vi "Method Elements.vi"(6 "Arduino In":cluster{"Error In":errorcluster, "LINX In":T1}, 7 "Potential Calibration":dbl[][](array[numeric])=[[1.0, 0.0, 5.4592, 5.4592]], 8 "Input--Scan Rate":cluster{"DE (V)":dbl, "Dt (s)":dbl}={"DE (V)"=1.0, "Dt (s)"=1.0} {"Dt (s)" format="%0.2f"; "DE (V)" format="%0.2f"}, 9 "Input--Timing":T9={"Duration (s)"=30.0, "Sample Rate (ms)"=100.0, "Frequency (mHz)"=1000.0, "Repeat n Times"=0}, 10 "Input--Potential":T8={"Ei (V)"=0.0, "Ef (V)"=1.0, "E1 (V)"=1.0, "E2 (V)"=-1.0, "Duty Cycle (%)"=50.0}, 11 "Element":T10(ring)) -> (3 "Output":T7, 4 "Arduino Out":cluster{"Error Out":errorcluster, "LINX Out":T1})   [LabVIEW 2022 SP3]
uses:
  <vilib>/MakerHub/LINX/Private/Type Defs/LINX Ref.ctl
  <vilib>/MakerHub/LINX/Private/Type Defs/Platform.ctl
  <vilib>/MakerHub/LINX/Private/Type Defs/Interface.ctl
  <vilib>/MakerHub/LINX/Private/Device/Type Defs/LINX Device Config.ctl
  <vilib>/MakerHub/LINX/Private/Device/Type Defs/TCP Config.ctl
  <vilib>/MakerHub/LINX/Private/Device/Type Defs/Channels.ctl
  <vilib>/Analysis/1siggen.llb/Ramp Pattern by Samples.vi
  <vilib>/Analysis/NI_AALBase.lvlib
  <vilib>/MakerHub/LINX/LMH-LINX.lvlib
  <vilib>/MakerHub/LINX/Private/Device/Device.lvlib
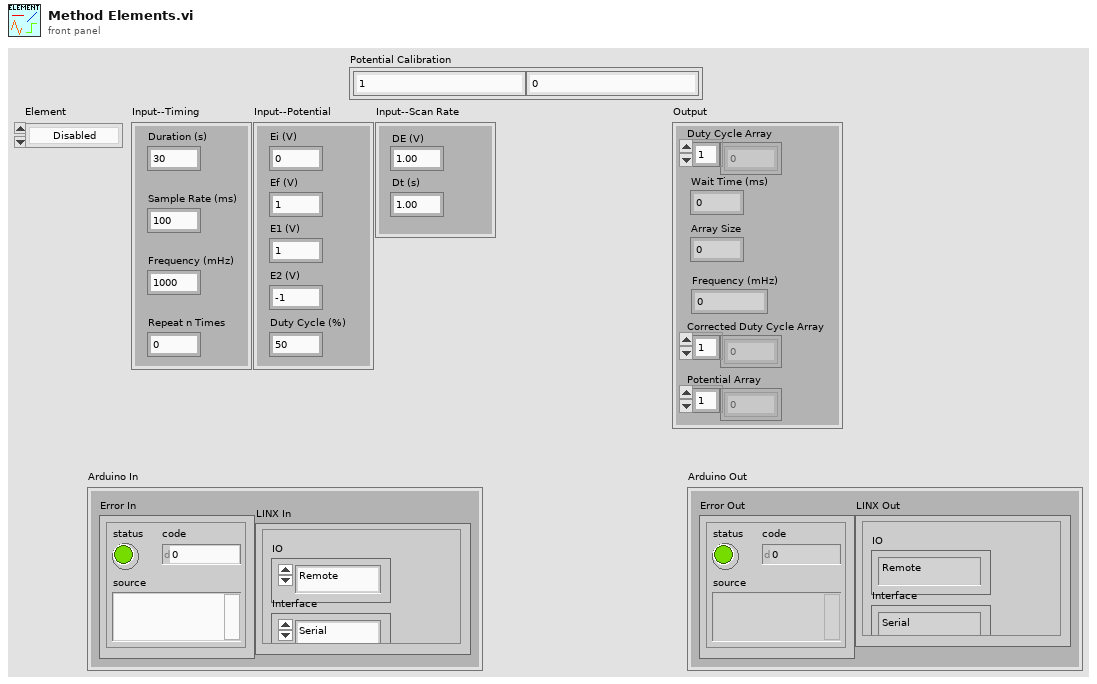
[diagram p1: front panel]
types:
  T1 = typedef "LMH-LINX.lvlib/LINX Ref.ctl" = cluster{"IO":T2, "Interface":T3, "LINX Device Config":T4}
  T2 = typedef "LMH-LINX.lvlib/Platform.ctl" = enum16{"Remote", "Local"}
  T3 = typedef "LMH-LINX.lvlib/Interface.ctl" = enum16{"Serial", "TCP"}
  T4 = typedef "LMH-LINX.lvlib/Device.lvlib/LINX Device Config.ctl" = cluster{"Interface":T3, "COM Port":refnum<visa-resource-name>, "TCP Configuration":T5, "Device Family":u8, "Device ID":u8, "Device Name":string, "TCP Ref":refnum<k5>, "Channels":T6}
  T5 = typedef "LMH-LINX.lvlib/Device.lvlib/TCP Config.ctl" = cluster{"IP Address":string, "Port":u16}
  T6 = typedef "LMH-LINX.lvlib/Channels.ctl" = cluster{"DI":u8[], "DO":u8[], "AI":u8[], "AO":u8[], "PWM":u8[], "QE":u8[], "UART":u8[], "I2C 2":u8[], "SPI":u8[], "CAN":u8[], "Servo":u8[], "AI Ref (V)":dbl, "AI Resolution (Bits)":u8, "AO Ref (V)":dbl, "AO Resolution (Bits)":u8}
  T7 = cluster{"Duty Cycle Array":dbl[], "Wait Time (ms)":dbl, "Array Size":i32, "Frequency (mHz)":dbl, "Corrected Duty Cycle Array":dbl[], "Potential Array":dbl[]}
  T8 = cluster{"Ei (V)":dbl, "Ef (V)":dbl, "E1 (V)":dbl, "E2 (V)":dbl, "Duty Cycle (%)":dbl}
  T9 = cluster{"Duration (s)":dbl, "Sample Rate (ms)":dbl, "Frequency (mHz)":dbl, "Repeat n Times":i32}
  T10 = enum16{"Disabled", "Potentiostatic", "Linear Ramp", "Staircase Ramp", "Triangle Wave", "Square Wave", "Staircase Wave", "Sine Wave"}
  T11 = cluster{dbl[], "Sample Rate (ms)":dbl, i32, "Frequency (mHz)":dbl, dbl[], "Ramp Pattern":dbl[]}
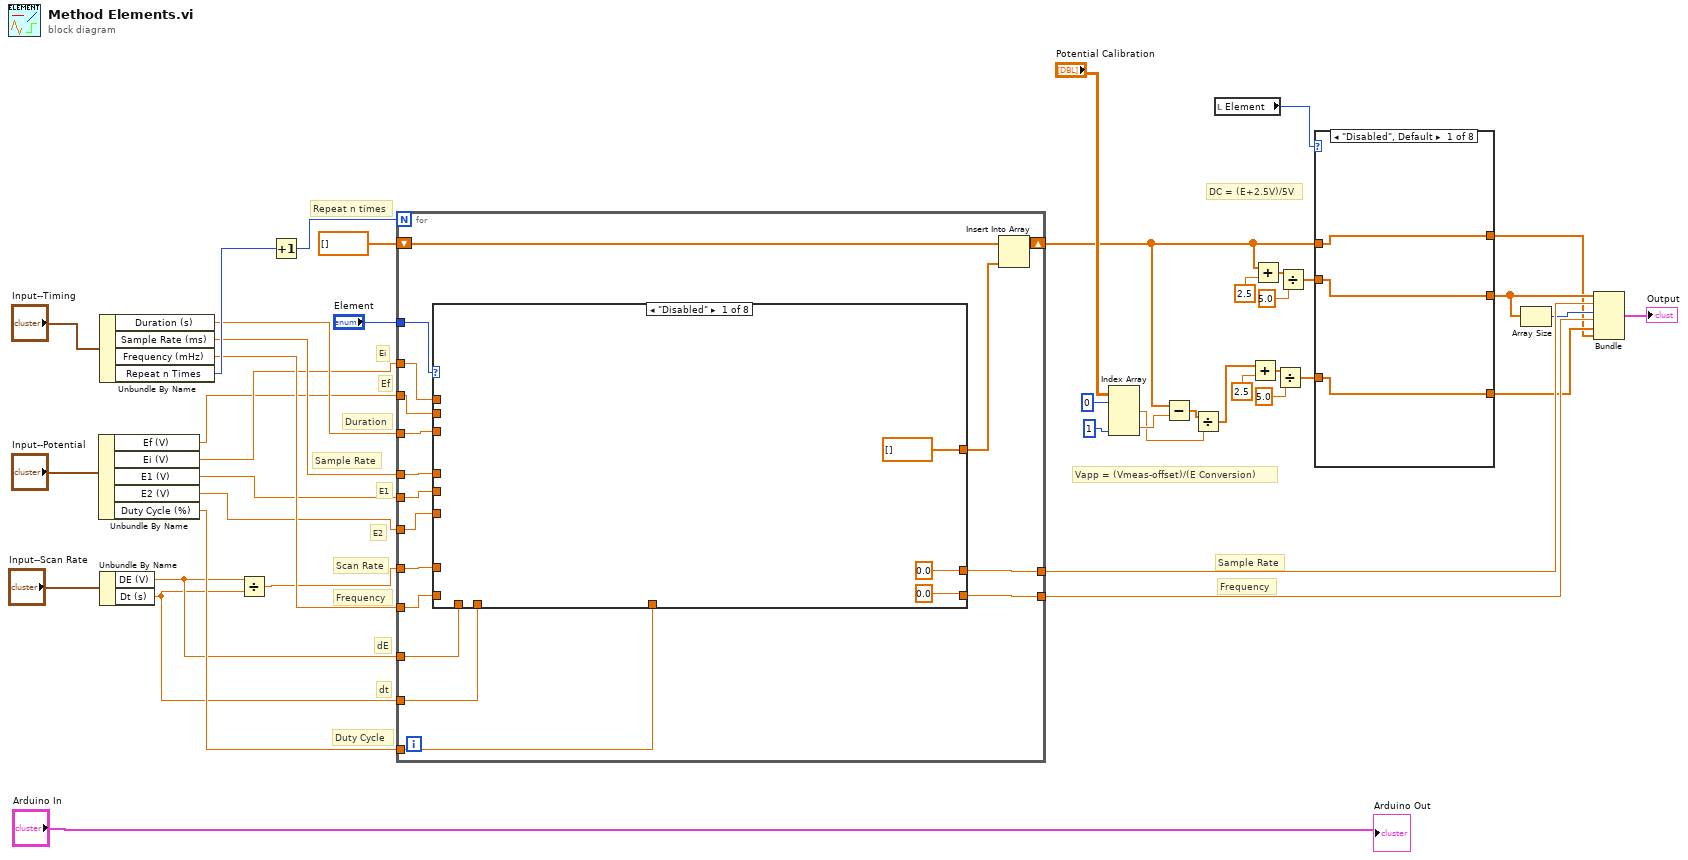
[diagram p0: block diagram]
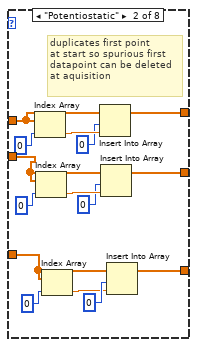
[diagram p2: hidden frame]
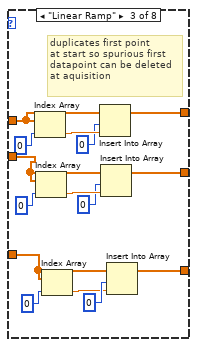
[diagram p3: hidden frame]
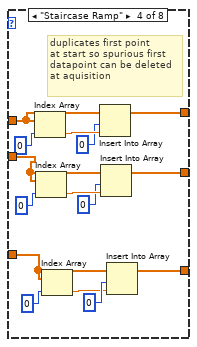
[diagram p4: hidden frame]
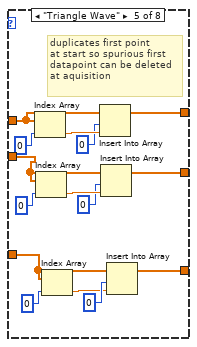
[diagram p5: hidden frame]
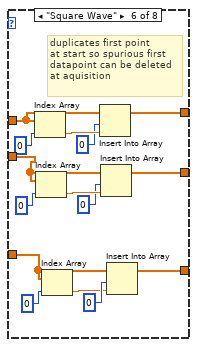
[diagram p6: hidden frame]
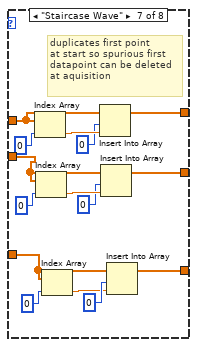
[diagram p7: hidden frame]
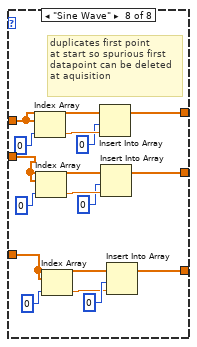
[diagram p8: hidden frame]
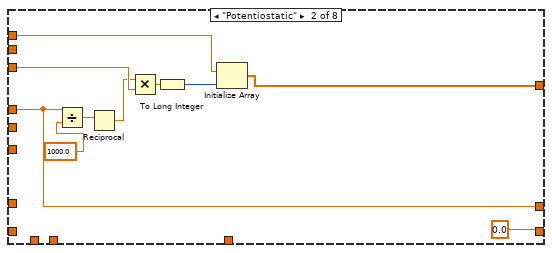
[diagram p9: hidden frame]
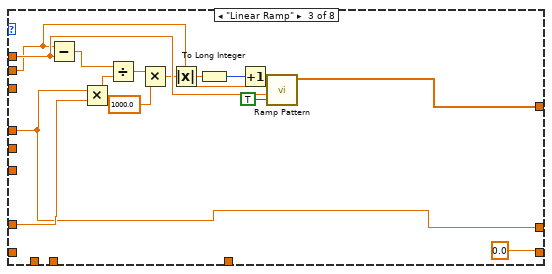
[diagram p10: hidden frame]
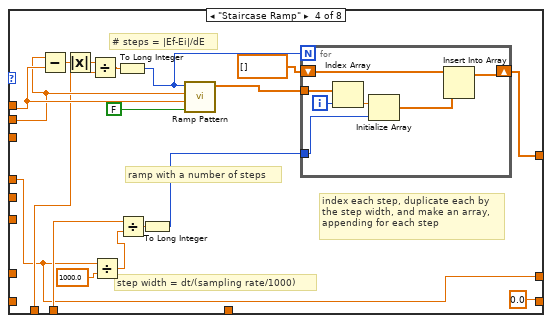
[diagram p11: hidden frame]
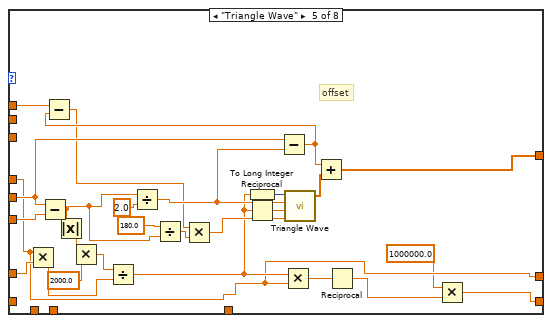
[diagram p12: hidden frame]
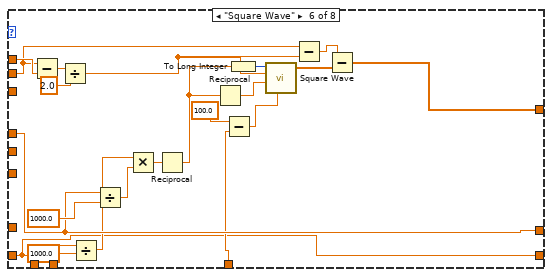
[diagram p13: hidden frame]
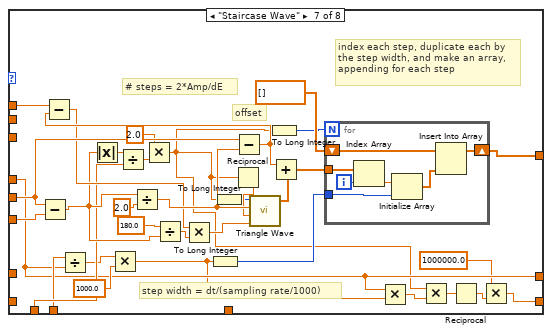
[diagram p14: hidden frame]
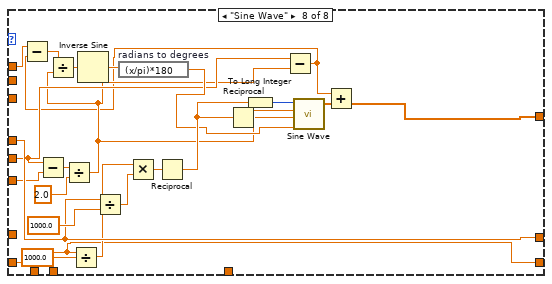
[diagram p15: hidden frame]
diagram:
  w7 = 0 ("index")
  # "Vapp = (Vmeas-offset)/(E Conversion)"
  # "DC = (E+2.5V)/5V"
  # "Frequency"
  # "Sample Rate"
  # "Repeat n times"
  # "dt"
  # "dE"
  # "Duty Cycle"
  # "Frequency"
  # "E2"
  # "E1"
  # "Ef"
  # "Ei"
  # "Sample Rate"
  # "Duration"
  # "Scan Rate"
  n1 = Unbundle By Name("Input--Potential") -> ("Ef (V)"=w27:dbl, "Ei (V)"=w28:dbl, "E1 (V)"=w26:dbl, "E2 (V)"=w25:dbl, "Duty Cycle (%)"=w24:dbl)
  n2 = Unbundle By Name("Input--Timing") -> ("Duration (s)"=w30:dbl, "Sample Rate (ms)"=w31:dbl, "Frequency (mHz)"=w32:dbl, "Repeat n Times"=w33:i32)
  n3 = Unbundle By Name("Input--Scan Rate") -> ("DE (V)"=w22:dbl, "Dt (s)"=w20:dbl)
  n4 = Divide(x=w22, y=w20) -> (x/y=w21:dbl)
  n5 = Increment(x=w33) -> (x+1=w37:i32)
  n6 = for {
    N: w37 -> [_]
    tunnel: "Element" -> [w60]
    tunnel: w30 -> [w59]
    tunnel: w24 -> [w58]
    tunnel: w28 -> [w57]
    tunnel: w27 -> [w56]
    tunnel: w26 -> [w55]
    tunnel: w25 -> [w46]
    tunnel: w32 -> [w54]
    tunnel: w21 -> [w53]
    tunnel: w31 -> [w52]
    tunnel: [w51] -> w39
    tunnel: [w50] -> w38
    shift-right: [w47] -> w3
    shift-left: dbl[] [] ("Ramp Pattern") -> [w48]
    tunnel: w22 -> [w45]
    tunnel: w20 -> [w44]
    n7 = case shown="\"Disabled\"" w60 {
      tunnel: w59 -> [_ w72 _ _ _ _ _ _]
      tunnel: w57 -> [_ w73 w84 w96 w135 w159 w190 w207]
      tunnel: w56 -> [_ _ w83 w95 _ w156 _ _]
      tunnel: w53 -> [_ _ w88 _ w127 _ _ _]
      tunnel: w55 -> [_ _ _ _ w137 _ w192 w210]
      tunnel: w46 -> [_ _ _ _ w139 _ w194 w211]
      tunnel: [0.0 ("Sampling Rate (ms)") w71 w80 w91 w119 w149 w170 w220] -> w51
      tunnel: w52 -> [_ w71 w80 w91 w119 w149 w170 w220]
      tunnel: w58 -> [_ _ _ _ _ w144 _ _]
      tunnel: w54 -> [_ _ _ _ _ w142 _ w205]
      tunnel: [0.0 ("Frequency (mHz)") 0.0 ("Frequency (Hz)") 0.0 ("Frequency (Hz)") 0.0 ("Frequency (mHz)") w116 w142 w163 w205] -> w50
      tunnel: [dbl[] [] ("Ramp Pattern") w65 w77 w90 w128 w146 w177 w204] -> w49
      tunnel: w45 -> [_ _ _ w94 _ _ w182 _]
      tunnel: w44 -> [_ _ _ w93 _ _ w175 _]
      frame "Disabled" {
      }
      frame "Potentiostatic" {
        n8 = Divide(x=w71, y=1000.0) -> (x/y=w67:dbl)
        n9 = Reciprocal(x=w67) -> (1/x=w69:dbl)
        n10 = Multiply(x=w69, y=w72) -> (x*y=w68:dbl)
        n11 = To Long Integer(number=w68) -> (32bit integer=w64:i32)
        n12 = Initialize Array(w73, w64) -> (w65:dbl[])
      }
      frame "Linear Ramp" {
        n13 = Subtract(x=w83, y=w84) -> (x-y=w86:dbl)
        n14 = Multiply(x=w80, y=w88) -> (x*y=w87:dbl)
        n15 = Divide(x=w86, y=w87) -> (x/y=w85:dbl)
        n16 = Multiply(x=w85, y=1000.0) -> (x*y=w82:dbl)
        n17 = Absolute Value(x=w82) -> (abs(x)=w79:dbl)
        n18 = To Long Integer(number=w79) -> (32bit integer=w76:i32)
        n19 = Increment(x=w76) -> (x+1=w75:i32)
        n20 = call-poly <vilib>:"Ramp Pattern.vi"("exclude end?"=TRUE, "start"=w84, "end"=w83, "samples"=w75) -> ("Ramp Pattern"=w77:dbl[])  [unwired: 6 in, 1 out]
      }
      frame "Staircase Ramp" {
        # "index each step, duplicate each by\nthe step width, and make an array,\nappending for each step"
        # "step width = dt/(sampling rate/1000)"
        # "# steps = |Ef-Ei|/dE"
        # "ramp with a number of steps"
        n21 = Subtract(x=w95, y=w96) -> (x-y=w100:dbl)
        n22 = Absolute Value(x=w100) -> (abs(x)=w106:dbl)
        n23 = Divide(x=w106, y=w94) -> (x/y=w101:dbl)
        n24 = Divide(x=w91, y=1000.0) -> (x/y=w103:dbl)
        n25 = To Long Integer(number=w101) -> (32bit integer=w105:i32)
        n26 = Divide(x=w93, y=w103) -> (x/y=w102:dbl)
        n27 = To Long Integer(number=w102) -> (32bit integer=w104:i32)
        n28 = call-poly <vilib>:"Ramp Pattern.vi"("exclude end?"=FALSE, "start"=w96, "end"=w95, "samples"=w105) -> ("Ramp Pattern"=w99:dbl[])  [unwired: 6 in, 1 out]
        n29 = for {
          N: w105 -> [_]
          tunnel: w99 -> [w112]
          tunnel: w104 -> [w110]
          shift-right: [w109] -> w90
          shift-left: dbl[] [] -> [w108]
          i -> [w113]
          n30 = Index Array(array=w112, index=w113) -> (element=w111:dbl)
          n31 = Initialize Array(w111, w110) -> (w107:dbl[])
          n32 = Insert Into Array(array=w108, new element=w107) -> (w109:dbl[])  [unwired: 1 in]
        }
      }
      frame "Triangle Wave" {
        # "offset"
        n33 = Multiply(x=w119, y=w127) -> (x*y=w123:dbl)
        n34 = Subtract(x=w137, y=w139) -> (x-y=w126:dbl)
        n35 = Absolute Value(x=w126) -> (abs(x)=w118:dbl)
        n36 = Multiply(x=w118, y=2000.0) -> (x*y=w124:dbl)
        n37 = Divide(x=w124, y=w123) -> (x/y=w122:dbl)
        n38 = Divide(x=w126, y=2.0) -> (x/y=w133:dbl)
        n39 = Divide(x=180.0, y=w126) -> (x/y=w131:dbl)
        n40 = To Long Integer(number=w122) -> (32bit integer=w114:i32)
        n41 = Reciprocal(x=w122) -> (1/x=w121:dbl)
        n42 = Subtract(x=w137, y=w133) -> (x-y=w134:dbl)
        n43 = Subtract(x=w135, y=w134) -> (x-y=w129:dbl)
        n44 = Multiply(x=w129, y=w131) -> (x*y=w130:dbl)
        n45 = Multiply(x=w122, y=w119) -> (x*y=w120:dbl)
        n46 = call <vilib>:"Triangle Wave.vi"("samples"=w114, "amplitude"=w133, "frequency"=w121, "phase in"=w130) -> ("triangle wave"=w136:dbl[])  [unwired: 1 in, 2 out]
        n47 = Add(x=w134, y=w136) -> (x+y=w128:dbl[])
        n48 = Reciprocal(x=w120) -> (1/x=w115:dbl)
        n49 = Multiply(x=1000000.0, y=w115) -> (x*y=w116:dbl)
      }
      frame "Square Wave" {
        n50 = Subtract(x=w156, y=w159) -> (x-y=w158:dbl)
        n51 = Divide(x=w158, y=2.0) -> (x/y=w155:dbl)
        n52 = Divide(x=w142, y=1000.0) -> (x/y=w148:dbl)
        n53 = Divide(x=w149, y=1000.0) -> (x/y=w153:dbl)
        n54 = Multiply(x=w148, y=w153) -> (x*y=w152:dbl)
        n55 = Reciprocal(x=w152) -> (1/x=w151:dbl)
        n56 = Reciprocal(x=w151) -> (1/x=w141:dbl)
        n57 = Subtract(x=100.0, y=w144) -> (x-y=w143:dbl)
        n58 = To Long Integer(number=w151) -> (32bit integer=w140:i32)
        n59 = call <vilib>:"Square Wave.vi"("samples"=w140, "amplitude"=w155, "frequency"=w141, "duty cycle (%)"=w143) -> ("square wave"=w150:dbl[])  [unwired: 2 in, 2 out]
        n60 = Subtract(x=w156, y=w155) -> (x-y=w154:dbl)
        n61 = Subtract(x=w154, y=w150) -> (x-y=w146:dbl[])
      }
      frame "Staircase Wave" {
        # "step width = dt/(sampling rate/1000)"
        # "# steps = 2*Amp/dE"
        # "index each step, duplicate each by\nthe step width, and make an array,\nappending for each step"
        # "offset"
        n62 = Subtract(x=w192, y=w194) -> (x-y=w183:dbl)
        n63 = Divide(x=w175, y=w170) -> (x/y=w173:dbl)
        n64 = Absolute Value(x=w183) -> (abs(x)=w181:dbl)
        n65 = Multiply(x=w173, y=1000.0) -> (x*y=w169:dbl)
        n66 = Divide(x=w181, y=w182) -> (x/y=w180:dbl)
        n67 = Divide(x=w183, y=2.0) -> (x/y=w188:dbl)
        n68 = Multiply(x=2.0, y=w180) -> (x*y=w167:dbl)
        n69 = Divide(x=180.0, y=w183) -> (x/y=w186:dbl)
        n70 = To Long Integer(number=w169) -> (32bit integer=w172:i32)
        n71 = To Long Integer(number=w167) -> (32bit integer=w162:i32)
        n72 = Reciprocal(x=w167) -> (1/x=w171:dbl)
        n73 = Subtract(x=w192, y=w188) -> (x-y=w189:dbl)
        n74 = Subtract(x=w190, y=w189) -> (x-y=w184:dbl)
        n75 = Multiply(x=w184, y=w186) -> (x*y=w185:dbl)
        n76 = call <vilib>:"Triangle Wave.vi"("samples"=w162, "amplitude"=w188, "frequency"=w171, "phase in"=w185) -> ("triangle wave"=w191:dbl[])  [unwired: 1 in, 2 out]
        n77 = To Long Integer(number=w167) -> (32bit integer=w161:i32)
        n78 = Add(x=w189, y=w191) -> (x+y=w178:dbl[])
        n79 = for {
          N: w161 -> [_]
          tunnel: w178 -> [w200]
          shift-right: [w197] -> w177
          shift-left: dbl[] [] -> [w196]
          tunnel: w172 -> [w195]
          i -> [w201]
          n80 = Index Array(array=w200, index=w201) -> (element=w199:dbl)
          n81 = Initialize Array(w199, w195) -> (w198:dbl[])
          n82 = Insert Into Array(array=w196, new element=w198) -> (w197:dbl[])  [unwired: 1 in]
        }
        n83 = Multiply(x=w170, y=w169) -> (x*y=w168:dbl)
        n84 = Multiply(x=w167, y=w168) -> (x*y=w166:dbl)
        n85 = Reciprocal(x=w166) -> (1/x=w165:dbl)
        n86 = Multiply(x=1000000.0, y=w165) -> (x*y=w163:dbl)
      }
      frame "Sine Wave" {
        n87 = Subtract(x=w210, y=w211) -> (x-y=w215:dbl)
        n88 = Divide(x=w215, y=2.0) -> (x/y=w209:dbl)
        n89 = Divide(x=w205, y=1000.0) -> (x/y=w219:dbl)
        n90 = Divide(x=w220, y=1000.0) -> (x/y=w223:dbl)
        n91 = Multiply(x=w219, y=w223) -> (x*y=w222:dbl)
        n92 = Reciprocal(x=w222) -> (1/x=w221:dbl)
        n93 = Reciprocal(x=w221) -> (1/x=w203:dbl)
        n94 = To Long Integer(number=w221) -> (32bit integer=w202:i32)
        n95 = Subtract(x=w210, y=w209) -> (x-y=w206:dbl)
        n96 = Subtract(x=w207, y=w206) -> (x-y=w208:dbl)
        n97 = Divide(x=w208, y=w209) -> (x/y=w214:dbl)
        n98 = Inverse Sine(1:w214) -> (0:w213:dbl)
        n99 = expression code="(x/pi)*180" "radians to degrees"(w213) -> (w212:dbl)
        n100 = call <vilib>:"Sine Wave.vi"("samples"=w202, "amplitude"=w209, "frequency"=w203, "phase in"=w212) -> ("sine wave"=w216:dbl[])  [unwired: 1 in, 2 out]
        n101 = Add(x=w206, y=w216) -> (x+y=w204:dbl[])
      }
    }
    n102 = Insert Into Array(array=w48, new element=w49) -> (w47:dbl[])  [unwired: 1 in]
  }
  n103 = Index Array(array="Potential Calibration", index (row) #1=w7, index (col) #1=w7, index (row) #2=w7, index (col) #2=1 ("index")) -> (element #1=w5:dbl, element #2=w11:dbl)
  n104 = Subtract(x=w3, y=w11) -> (x-y=w10:dbl[])
  n105 = Divide(x=w10, y=w5) -> (x/y=w9:dbl[])
  n106 = local read "Element"() -> (w1:T10)
  n107 = Add(x=w9, y=2.5) -> (x+y=w12:dbl[])
  n108 = Add(x=w3, y=2.5) -> (x+y=w42:dbl[])
  n109 = Divide(x=w12, y=5.0) -> (x/y=w15:dbl[])
  n110 = Divide(x=w42, y=5.0) -> (x/y=w18:dbl[])
  n111 = case shown="\"Disabled\", Default" w1 {
    tunnel: w18 -> [w226 w239 w254 w269 w284 w299 w314 w329]
    tunnel: [w226 w238 w253 w268 w283 w298 w313 w328] -> w17
    tunnel: w15 -> [w225 w237 w252 w267 w282 w297 w312 w327]
    tunnel: [w225 w233 w248 w263 w278 w293 w308 w323] -> w4
    tunnel: w3 -> [w227 w229 w244 w259 w274 w289 w304 w319]
    tunnel: [w227 w228 w243 w258 w273 w288 w303 w318] -> w2
    frame "Disabled", Default {
    }
    frame "Potentiostatic" {
      # "duplicates first point\nat start so spurious first\ndatapoint can be deleted\nat aquisition"
      n112 = Index Array(array=w229, index=0) -> (element=w231:dbl)
      n113 = Index Array(array=w239, index=0) -> (element=w241:dbl)
      n114 = Index Array(array=w237, index=0) -> (element=w235:dbl)
      n115 = Insert Into Array(array=w229, index=0, new element=w231) -> (w228:dbl[])
      n116 = Insert Into Array(array=w239, index=0, new element=w241) -> (w238:dbl[])
      n117 = Insert Into Array(array=w237, index=0, new element=w235) -> (w233:dbl[])
    }
    frame "Linear Ramp" {
      # "duplicates first point\nat start so spurious first\ndatapoint can be deleted\nat aquisition"
      n118 = Index Array(array=w244, index=0) -> (element=w246:dbl)
      n119 = Index Array(array=w254, index=0) -> (element=w256:dbl)
      n120 = Index Array(array=w252, index=0) -> (element=w250:dbl)
      n121 = Insert Into Array(array=w244, index=0, new element=w246) -> (w243:dbl[])
      n122 = Insert Into Array(array=w254, index=0, new element=w256) -> (w253:dbl[])
      n123 = Insert Into Array(array=w252, index=0, new element=w250) -> (w248:dbl[])
    }
    frame "Staircase Ramp" {
      # "duplicates first point\nat start so spurious first\ndatapoint can be deleted\nat aquisition"
      n124 = Index Array(array=w259, index=0) -> (element=w261:dbl)
      n125 = Index Array(array=w269, index=0) -> (element=w271:dbl)
      n126 = Index Array(array=w267, index=0) -> (element=w265:dbl)
      n127 = Insert Into Array(array=w259, index=0, new element=w261) -> (w258:dbl[])
      n128 = Insert Into Array(array=w269, index=0, new element=w271) -> (w268:dbl[])
      n129 = Insert Into Array(array=w267, index=0, new element=w265) -> (w263:dbl[])
    }
    frame "Triangle Wave" {
      # "duplicates first point\nat start so spurious first\ndatapoint can be deleted\nat aquisition"
      n130 = Index Array(array=w274, index=0) -> (element=w276:dbl)
      n131 = Index Array(array=w284, index=0) -> (element=w286:dbl)
      n132 = Index Array(array=w282, index=0) -> (element=w280:dbl)
      n133 = Insert Into Array(array=w274, index=0, new element=w276) -> (w273:dbl[])
      n134 = Insert Into Array(array=w284, index=0, new element=w286) -> (w283:dbl[])
      n135 = Insert Into Array(array=w282, index=0, new element=w280) -> (w278:dbl[])
    }
    frame "Square Wave" {
      # "duplicates first point\nat start so spurious first\ndatapoint can be deleted\nat aquisition"
      n136 = Index Array(array=w289, index=0) -> (element=w291:dbl)
      n137 = Index Array(array=w299, index=0) -> (element=w301:dbl)
      n138 = Index Array(array=w297, index=0) -> (element=w295:dbl)
      n139 = Insert Into Array(array=w289, index=0, new element=w291) -> (w288:dbl[])
      n140 = Insert Into Array(array=w299, index=0, new element=w301) -> (w298:dbl[])
      n141 = Insert Into Array(array=w297, index=0, new element=w295) -> (w293:dbl[])
    }
    frame "Staircase Wave" {
      # "duplicates first point\nat start so spurious first\ndatapoint can be deleted\nat aquisition"
      n142 = Index Array(array=w304, index=0) -> (element=w306:dbl)
      n143 = Index Array(array=w314, index=0) -> (element=w316:dbl)
      n144 = Index Array(array=w312, index=0) -> (element=w310:dbl)
      n145 = Insert Into Array(array=w304, index=0, new element=w306) -> (w303:dbl[])
      n146 = Insert Into Array(array=w314, index=0, new element=w316) -> (w313:dbl[])
      n147 = Insert Into Array(array=w312, index=0, new element=w310) -> (w308:dbl[])
    }
    frame "Sine Wave" {
      # "duplicates first point\nat start so spurious first\ndatapoint can be deleted\nat aquisition"
      n148 = Index Array(array=w319, index=0) -> (element=w321:dbl)
      n149 = Index Array(array=w329, index=0) -> (element=w331:dbl)
      n150 = Index Array(array=w327, index=0) -> (element=w325:dbl)
      n151 = Insert Into Array(array=w319, index=0, new element=w321) -> (w318:dbl[])
      n152 = Insert Into Array(array=w329, index=0, new element=w331) -> (w328:dbl[])
      n153 = Insert Into Array(array=w327, index=0, new element=w325) -> (w323:dbl[])
    }
  }
  n154 = Array Size(array=w17) -> (size(s)=w35:i32)
  n155 = Bundle(w17, "Sample Rate (ms)"=w39, w35, "Frequency (mHz)"=w38, w4, "Ramp Pattern"=w2) -> (→"Output":T11)  [unwired: 1 in]
  "Arduino Out" <- "Arduino In"
